vi "Connect Error Wires.vi"(0 "node in":refnum<vi>, 5 "new object ref":refnum<vi>, 9 "string":string, 11 "error in":errorcluster) -> (15 "error out":errorcluster)   [LabVIEW 2021, in "Converter.lvlib"]
uses:
  Converter.lvlib
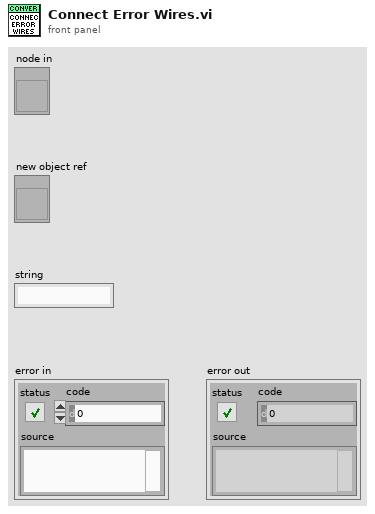
[diagram p1: front panel]
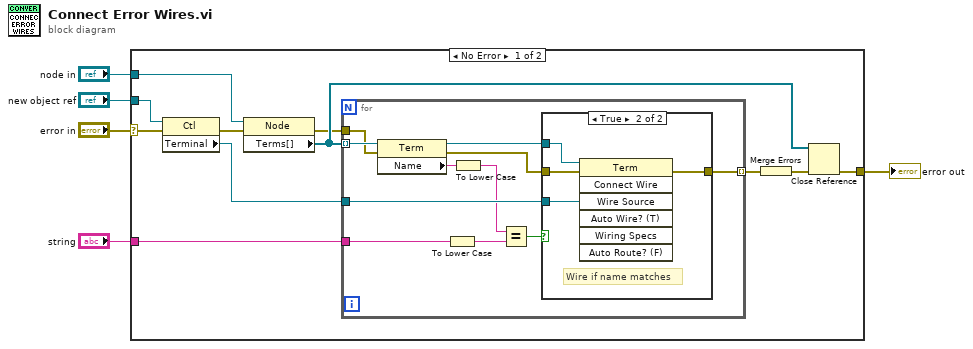
[diagram p0: block diagram]
diagram:
  n1 = case shown="No Error" "error in" {
    selector: "error in" -> [w15 w33]
    tunnel: "new object ref" -> [w13 _]
    tunnel: [w11 w33] -> w3
    tunnel: "node in" -> [w7 _]
    tunnel: "string" -> [w6 _]
    frame No Error {
      n2 = property class="Ctl"(reference=w13, error in=w15) -> (error out=w14:errorcluster, "Terminal"=w16:refnum<vi>)  [unwired: 1 out]
      n3 = property class="Node"(reference=w7, error in=w14) -> (error out=w8:errorcluster, "Terms[]"=w12:refnum<vi>[])  [unwired: 1 out]
      n4 = for {
        tunnel: w12 -> [w27] mode=indexing
        tunnel: w8 -> [w26]
        tunnel: w6 -> [w24]
        tunnel: [w20] -> w9 mode=indexing
        tunnel: w16 -> [w19]
        n5 = property class="Term"(reference=w27, error in=w26) -> (reference out=w21:refnum<vi>, error out=w22:errorcluster, "Name"=w25:string)
        n6 = To Lower Case(string=w24) -> (all lower case string=w17:string)
        n7 = To Lower Case(string=w25) -> (all lower case string=w18:string)
        n8 = Equal?(x=w18, y=w17) -> (x = y?=w23:bool)
        n9 = case shown="True" w23 {
          tunnel: w22 -> [w28 w32]
          tunnel: w21 -> [_ w31]
          tunnel: [w28 w30] -> w20
          tunnel: w19 -> [_ w29]
          frame False {
          }
          frame True {
            # "Wire if name matches"
            n10 = invoke class="Term" method="Connect Wire"(reference=w31, error in=w32, "Wire Source"=w29) -> (error out=w30:errorcluster)  [unwired: 4 in, 6 out]
          }
        }
      }
      n11 = Merge Errors(w9) -> (w10:errorcluster)
      n12 = Close Reference(reference=w12, error in (no error)=w10) -> (error out=w11:errorcluster)
    }
    frame Error {
    }
  }
  "error out" <- w3
